vi "Acquisition Done.vi"(8 "error in (no error)":errorcluster, 11 "Camera_Scan_Controller.lvclass":refnum<class "Camera_Scan_Controller.lvclass">) -> (0 "error out":errorcluster, 3 "Camera_Scan_Controller.lvlib:Camera_Scan_Controller.lvclass":refnum<class "Camera_Scan_Controller.lvclass">)   [LabVIEW 2023, in "Camera_Scan_Controller.lvlib" / "Camera_Scan_Controller.lvclass"]
uses:
  Camera_Scan_Controller.lvclass
  Camera_Scan_Controller.lvclass/Camera_Scan_Controller.ctl
  <vilib>/ActorFramework/Message Enqueuer/Message Enqueuer.lvclass/Message Enqueuer.ctl
  <vilib>/ActorFramework/Message Enqueuer/Enqueue.vi
  UIs/Camera_Controller/Camera_Controller/TopControllerComm Messages/External_Move Msg/External_Move Msg.lvclass
  C:/Program Files/National Instruments/LabVIEW 2023/vi.lib/ActorFramework/Message/Message.lvclass
  UIs/Camera_Controller/Camera_Controller/TopControllerComm Messages/ScanDone Msg/ScanDone Msg.lvclass
  <vilib>/ActorFramework/Message Priority Queue/Priority Enqueue.vi
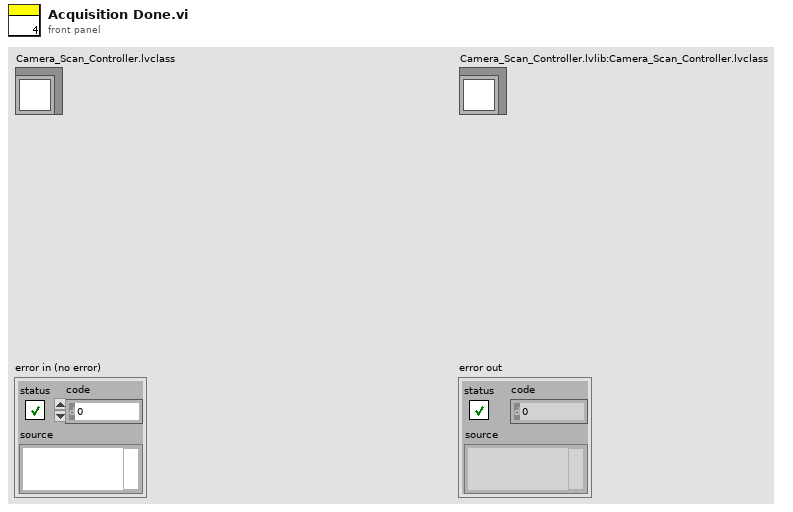
[diagram p1: front panel]
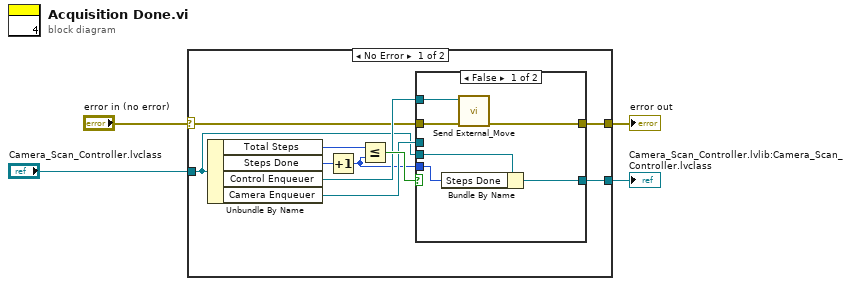
[diagram p0: block diagram]
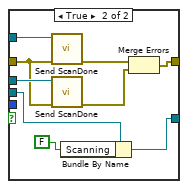
[diagram p2: hidden frame]
diagram:
  n1 = case shown="No Error" "error in (no error)" {
    selector: "error in (no error)" -> [w9 w31]
    tunnel: [w8 w31] -> w2
    tunnel: [w6 w30] -> w1
    tunnel: "Camera_Scan_Controller.lvclass" -> [w7 w30]
    frame No Error {
      n2 = Unbundle By Name(w7) -> ("Total Steps"=w13:u16, "Steps Done"=w14:u16, "Control Enqueuer"=w11:refnum<class "Message Enqueuer.lvclass">, "Camera Enqueuer"=w10:refnum<class "Message Enqueuer.lvclass">)
      n3 = Increment(x=w14) -> (x+1=w5:u16)
      n4 = Less Or Equal?(x=w13, y=w5) -> (x <= y?=w12:bool)
      n5 = case shown="False" w12 {
        tunnel: w11 -> [w17 w24]
        tunnel: w10 -> [_ w23]
        tunnel: w9 -> [w16 w22]
        tunnel: [w15 w29] -> w8
        tunnel: w7 -> [w20 w28]
        tunnel: [w18 w27] -> w6
        tunnel: w5 -> [w19 _]
        frame False {
          n6 = Bundle By Name(cluster=w20, "Steps Done"=w19) -> (w18:refnum<class "Camera_Scan_Controller.lvclass">)
          n7 = call "Send External_Move.vi"("error in (no error)"=w16, "Message Enqueuer"=w17) -> ("error out"=w15:errorcluster)  [unwired: 8 in, 1 out]
        }
        frame True {
          n8 = call "Send ScanDone.vi"("error in (no error)"=w22, "Message Enqueuer"=w24) -> ("error out"=w25:errorcluster)  [unwired: 8 in, 1 out]
          n9 = call "Send ScanDone.vi"("error in (no error)"=w22, "Message Enqueuer"=w23) -> ("error out"=w21:errorcluster)  [unwired: 8 in, 1 out]
          n10 = Bundle By Name(cluster=w28, "Scanning"=FALSE) -> (w27:refnum<class "Camera_Scan_Controller.lvclass">)
          n11 = Merge Errors(w25, w21) -> (w29:errorcluster)
        }
      }
    }
    frame Error {
    }
  }
  "error out" <- w2
  "Camera_Scan_Controller.lvlib:Camera_Scan_Controller.lvclass" <- w1
